vi "ParsePipeSeparatedList.vi"(11 "List":string) -> (3 "Array":string[](array[string]))   [LabVIEW 2017]
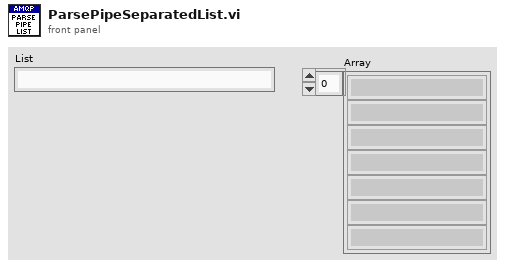
[diagram p1: front panel]
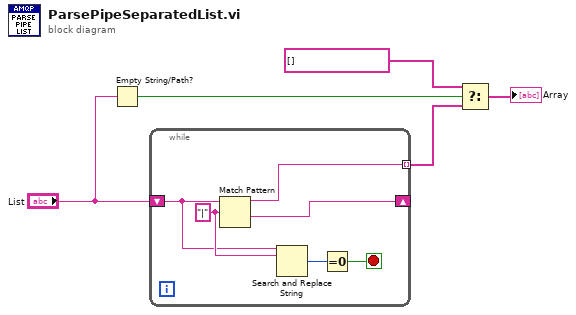
[diagram p0: block diagram]
diagram:
  n1 = Empty String/Path?(string/path="List") -> (empty?=w4:bool)
  n2 = while {
    tunnel: [w10] -> w3 mode=indexing
    shift-right: [w9] -> _
    shift-left: "List" -> [w6]
    stop <- w7 stop-if-true
    w11 = "|" ("regular expression")
    n3 = Match Pattern(string=w6, regular expression=w11) -> (before substring=w10:string, after substring=w9:string)  [unwired: 1 in, 2 out]
    n4 = Search and Replace String(input string=w6, search string=w11) -> (number of replacements=w8:i32)  [unwired: 6 in, 3 out]
    n5 = Equal To 0?(x=w8) -> (x = 0?=w7:bool)
  }
  n6 = Select(t=string[] [] ("s? t:f"), s=w4, f=w3) -> (s? t:f=→"Array":string[])
